vi "Stop or Error.vi"(1 "INSTR":u8, 6 "State In":T1, 8 "error in":errorcluster, 9 "Stop":bool) -> (0 "error out":errorcluster, 4 "State Out":T1)   [LabVIEW 2015]
uses:
  TypeDefs Host/States.ctl
  TypeDefs Host/Counter FGV Enum.ctl
  TypeDefs Host/Open Audio FGV Enum.ctl
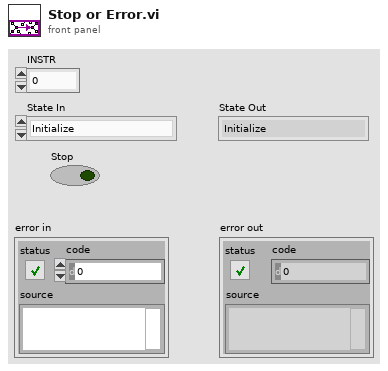
[diagram p1: front panel]
types:
  T1 = typedef "States.ctl" = enum16{"Initialize", "Calibrate", "Create", "Settings", "Shutdown"}
  T2 = typedef "Open Audio FGV Enum.ctl" = enum16{"Get", "Set"}
  T3 = typedef "Counter FGV Enum.ctl" = enum16{"Get Count", "Set Count"}
  T4 = typedef "Led Control.ctl" = enum32{"LED_OFF", "LED_GREEN", "LED_RED", "LED_YELLOW", "LED_BLINK_GREEN", "LED_BLINK_GREEN2", "LED_BLINK_RED_YELLOW"}
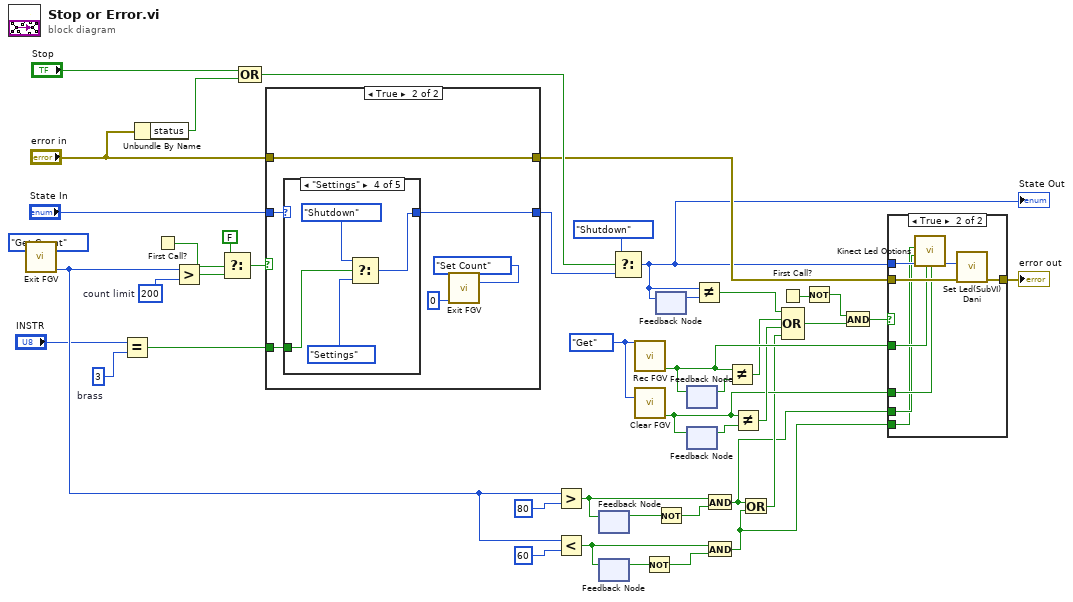
[diagram p0: block diagram]
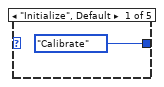
[diagram p4: hidden frame]
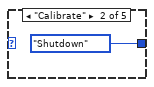
[diagram p5: hidden frame]
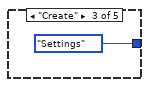
[diagram p6: hidden frame]
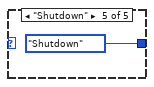
[diagram p7: hidden frame]
diagram:
  w2 = u8 3  # brass
  w24 = Open_Audio_FGV_Enum."Get" ("Command")
  w41 = i16 200  # count limit
  n1 = call "Exit FGV.vi"("Exit FGV Command"=Counter_FGV_Enum."Get Count") -> ("Count Out"=w9:i16)  [unwired: 10 in]
  n2 = Equal?(x="INSTR", y=w2) -> (x = y?=w1:bool)
  n3 = Unbundle By Name("error in") -> ("status"=w44:bool)
  n4 = First Call?() -> (First Call?: T/F=w40:bool)
  n5 = Greater?(x=w9, y=w41) -> (0:w39:bool)
  n6 = Select(t=FALSE, s=w40, f=w39) -> (s? t:f=w34:bool)
  n7 = Compound Arithmetic op=OR("Stop", w44) -> (w37:bool)
  n8 = case shown="True" w34 {
    tunnel: "State In" -> [w46 w52]
    tunnel: [w46 w50] -> w19
    tunnel: "error in" -> [w45 w49]
    tunnel: [w45 w49] -> w31
    tunnel: w1 -> [_ w47]
    frame False {
    }
    frame True {
      n9 = case shown="\"Settings\"" w52 {
        tunnel: [States."Calibrate" ("t") States."Shutdown" ("t") States."Settings" ("t") w56 States."Shutdown" ("t")] -> w50
        tunnel: w47 -> [_ _ _ w58 _]
        frame "Initialize", Default {
        }
        frame "Calibrate" {
        }
        frame "Create" {
        }
        frame "Settings" {
          n10 = Select(t=States."Shutdown", s=w58, f=States."Settings" ("t")) -> (s? t:f=w56:T1)
        }
        frame "Shutdown" {
        }
      }
      n11 = call "Exit FGV.vi"("Exit FGV Command"=Counter_FGV_Enum."Set Count", "Count In"=i16 0) -> ()  [unwired: 9 in, 1 out]
    }
  }
  n12 = Greater?(x=w9, y=i16 80) -> (0:w17:bool)
  n13 = Less?(x=w9, y=i16 60) -> (x < y?=w12:bool)
  n14 = feedback-in #1(w17) -> ()
  n15 = feedback #1() -> (w16:bool)  [unwired: 1 in]
  n16 = feedback #2() -> (w11:bool)  [unwired: 1 in]
  n17 = feedback-in #2(w12) -> ()
  n18 = Select(t=States."Shutdown", s=w37, f=w19) -> (s? t:f=w30:T1)
  "State Out" <- w30
  n19 = call "Rec FGV.vi"("Command"=w24) -> ("Rec?"=w25:bool)  [unwired: 10 in]
  n20 = call "Clear FGV.vi"("Command"=w24) -> ("Clear?"=w20:bool)  [unwired: 10 in]
  n21 = Not(x=w11) -> (.not. x?=w10:bool)
  n22 = feedback #3() -> (w32:T1)  [unwired: 1 in]
  n23 = feedback-in #3(w30) -> ()
  n24 = Not(x=w16) -> (.not. x?=w15:bool)
  n25 = feedback #4() -> (w26:bool)  [unwired: 1 in]
  n26 = feedback-in #4(w25) -> ()
  n27 = feedback #5() -> (w22:bool)  [unwired: 1 in]
  n28 = feedback-in #5(w20) -> ()
  n29 = Not Equal?(x=w30, y=w32) -> (x != y?=w27:bool)
  n30 = And(x=w17, y=w15) -> (x .and. y?=w8:bool)
  n31 = And(x=w12, y=w10) -> (x .and. y?=w7:bool)
  n32 = Not Equal?(x=w25, y=w26) -> (x != y?=w23:bool)
  n33 = Not Equal?(x=w20, y=w22) -> (x != y?=w21:bool)
  n34 = Or(x=w8, y=w7) -> (x .or. y?=w13:bool)
  n35 = First Call?() -> (First Call?: T/F=w28:bool)
  n36 = Compound Arithmetic op=OR(w27, w23, w21, w13) -> (w6:bool)
  n37 = Not(x=w28) -> (.not. x?=w4:bool)
  n38 = And(x=w4, y=w6) -> (x .and. y?=w5:bool)
  n39 = case shown="True" w5 {
    tunnel: [w61 w69] -> w29
    tunnel: w30 -> [_ w67]
    tunnel: w31 -> [w61 w66]
    tunnel: w25 -> [_ w65]
    tunnel: w20 -> [_ w64]
    tunnel: w8 -> [_ w63]
    tunnel: w7 -> [_ w62]
    frame False {
    }
    frame True {
      n40 = call "Kinect Led Options.vi"("Clear"=w64, "Rec"=w65, "States"=w67, "Bye active"=w63, "Bye inactive"=w62) -> ("Led Option"=w68:T4)  [unwired: 6 in]
      n41 = call "Set Led(SubVI) Dani.vi"("error in (no error)"=w66, "Led Option"=w68) -> ("error out"=w69:errorcluster)  [unwired: 9 in]
    }
  }
  "error out" <- w29
